vi "Find UUID.vi"(8 "error in (no error)":errorcluster, 10 "ID 2":u32, 11 "Data":T1[](array[typedef])) -> (0 "error out":errorcluster, 2 "Index":i32, 3 "dup Data":T1[](array[typedef]))   [LabVIEW 2014, in "Map Data.lvlib"]
doc: "Searches the data store for a single contact by ID."
uses:
  Map Data.lvlib
  MapDatas.ctl
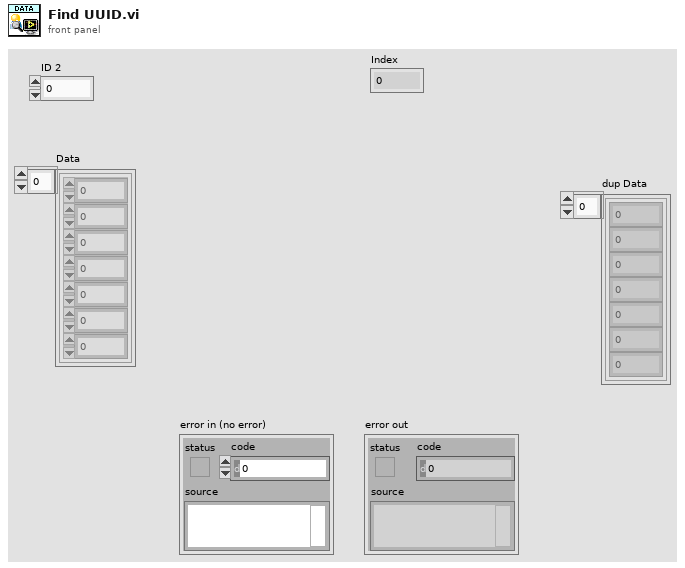
[diagram p1: front panel]
types:
  T1 = typedef "Map Data.lvlib/MapDatas.ctl" = cluster{"X":dbl, "Y":dbl, "Z":dbl, "heading":dbl, "X2":dbl, "Y2":dbl, "Z2":dbl}
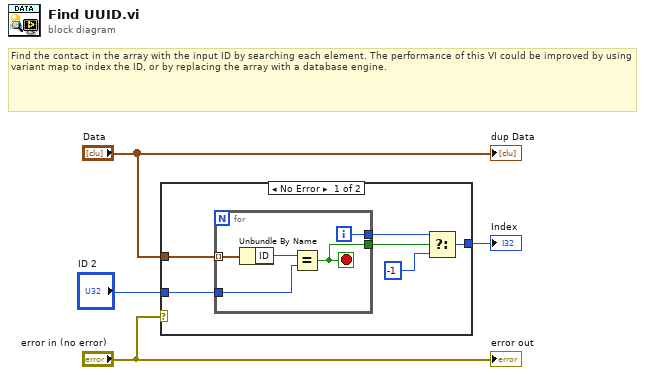
[diagram p0: block diagram]
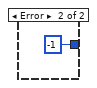
[diagram p2: hidden frame]
diagram:
  # "Find the contact in the array with the input ID by searching each element. The performance of this VI could be improved by using variant map to index the ID, or by replacing the array with a database engine."
  n1 = case shown="No Error" "error in (no error)" {
    tunnel: "ID 2" -> [w10 _]
    tunnel: "Data" -> [w9 _]
    tunnel: [w5 -1 ("f")] -> w3
    frame No Error {
      n2 = for {
        tunnel: w9 -> [w15] mode=indexing
        tunnel: w10 -> [w13]
        tunnel: [w12] -> w7
        tunnel: [w11] -> w8
        i -> [w12]
        stop <- w11 stop-if-true
        n3 = Unbundle By Name(w15) -> ("ID"=w14:u32)
        n4 = Equal?(x=w14, y=w13) -> (x = y?=w11:bool)
      }
      n5 = Select(t=w7, s=w8, f=-1) -> (s? t:f=w5:i32)
    }
    frame Error {
    }
  }
  "Index" <- w3
  "error out" <- "error in (no error)"
  "dup Data" <- "Data"
